vi "LinearControl.vi"(7 "SP_theta_e":dbl, 8 "Controller Gain":dbl[](array[numeric]) format="%.2f", 9 "setpoint":dbl) -> (1 "theta_e":dbl, 2 "pos":dbl)   [LabVIEW 2013]
uses:
  <vilib>/Simulation/ContinuousLinear/Implementation/NILVSim Derivative.llb/SIM derivative (scalar).vi
  <vilib>/Simulation/Implementation/XNodeFramework/SimXNode/SimX.xnode
  <vilib>/imath/engines/lvmath2/RunTimeEngine/NodeEndStatement/NIMS_NodeEndStatement_Output.vi
  <vilib>/imath/engines/lvmath2/RunTimeEngine/ErrorHandling/NIMS_Finalize Error.vi
  <vilib>/addons/Control Design/_Implementation/NI_CD_Implementation.lvlib
  <vilib>/addons/Control Design/_Implementation/CD State Feedback Controller (Single Output).vi
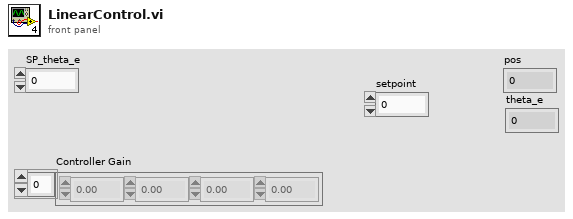
[diagram p1: front panel]
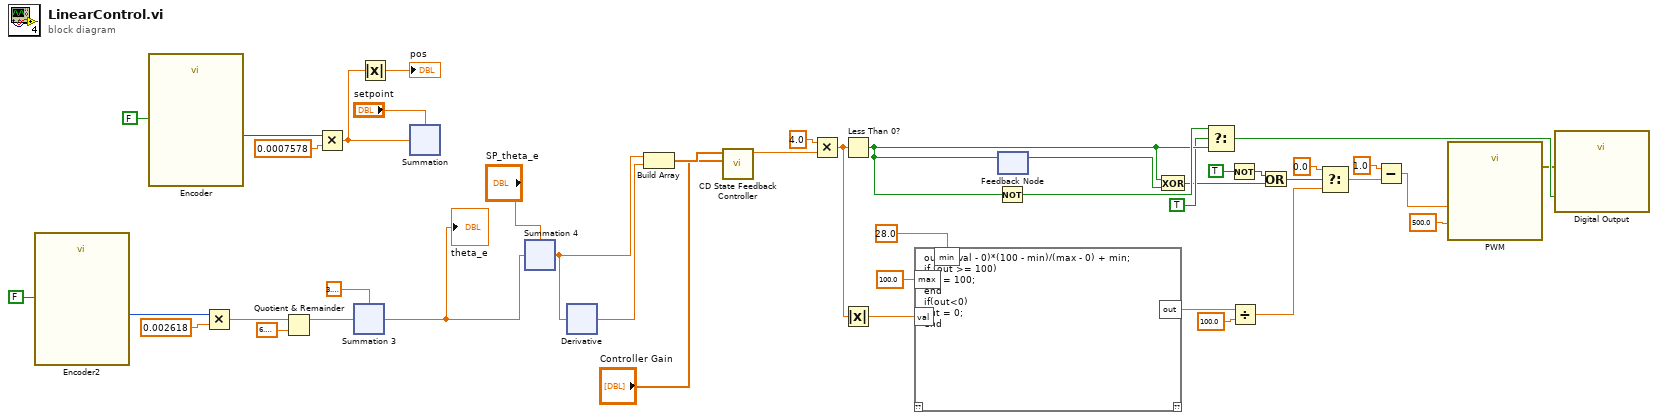
[diagram p0: block diagram]
diagram:
  n1 = call "Encoder2"("Reset Counter"=FALSE) -> ("Counter Value"=w40:i32)  [unwired: 23 in, 3 out]
  n2 = call "Encoder"("Reset Counter"=FALSE) -> ("Counter Value"=w42:i32)  [unwired: 23 in, 3 out]
  n3 = Multiply ("Multiply 3")(x=w40, y=0.002618 ("y 3")) -> (x*y=w37:dbl)
  n4 = Quotient & Remainder(x=w37, y=6.283185307179586 ("Constant 2")) -> (x-y*floor(x/y)=w36:dbl)  [unwired: 1 out]
  n5 = Multiply ("Multiply 2")(x=w42, y=0.0007578 ("y 2")) -> (x*y=w1:dbl)
  n6 = xnode "Summation 3"("Operand1"=3.141592653589793 ("Constant"), "Operand2"=w36) -> ("Result"=w3:dbl)
  "theta_e" <- w3
  n7 = Absolute Value(x=w1) -> (abs(x)=→"pos":dbl)
  n8 = xnode "Summation"("Operand1"="setpoint", "Operand2"=w1) -> ()  [unwired: 1 out]
  n9 = xnode "Summation 4"("Operand1"="SP_theta_e", "Operand2"=w3) -> ("Result"=w2:dbl)  [unwired: 1 in]
  n10 = xnode "Derivative"("input"=w2) -> ("output"=w32:dbl)  [unwired: 2 in]
  n11 = Build Array(w2, w32) -> (w10:dbl[])
  n12 = call-poly <vilib>:"CD State Feedback Controller.vi"("Controller Gain"="Controller Gain", "States"=w10) -> ("Controller Action"=w5:dbl)  [unwired: 8 in, 1 out]
  n13 = Multiply(x=4.0 ("x 2"), y=w5) -> (x*y=w6:dbl)
  n14 = Less Than 0?(x=w6) -> (x < 0?=w30:bool)
  n15 = Absolute Value ("Absolute Value 3")(x=w6) -> (abs(x)=w24:dbl)
  n16 = mathscript code="out = (val - 0)*(100 - min)/(max - 0) + min;\nif (out >= 100)\nout = 100;\nend\nif(out<0)\nout = 0;\nend"("val"=w24, "max"=100.0 ("max_in"), "min"=28.0 ("min_out")) -> ("out"=w26:dbl)  [unwired: 1 in, 1 out]
  n17 = Not ("Not 2")(x=w30) -> (.not. x?=w31:bool)
  n18 = feedback #1 ("Feedback Node 2")() -> (w19:bool)  [unwired: 1 in]
  n19 = feedback-in #1 ("3")(w30) -> ()
  n20 = Exclusive Or(1:w19, 2:w30) -> (0:w15:bool)
  n21 = Select ("Select 2")(t=w31, s=TRUE ("Inverted?"), f=w30) -> (s? t:f=w23:bool)
  n22 = Not(x=TRUE ("Enable")) -> (.not. x?=w16:bool)
  n23 = Divide(x=w26, y=100.0 ("y 4")) -> (x/y=w28:dbl)
  n24 = Or ("Or 2")(x=w16, y=w15) -> (x .or. y?=w18:bool)
  n25 = Select(t=0.0, s=w18, f=w28) -> (s? t:f=w14:dbl)
  n26 = Subtract(x=1.0, y=w14) -> (x-y=w21:dbl)
  n27 = call "PWM"("Duty Cycle (0-1)"=w21, "Frequency (Hz)"=500.0 ("pwm freq")) -> ("error out"=w11:errorcluster)  [unwired: 25 in]
  n28 = call "Digital Output"("A/DIO6 (Pin 23)"=w23, "error in (no error)"=w11) -> ()  [unwired: 25 in, 1 out]
